vi "Set Support Directory.vi"(8 "error in (no error)":errorcluster, 10 "Support Directory Path":path, 11 "ProjectItem in":refnum<vi>) -> (0 "error out":errorcluster, 3 "ProjectItem out":refnum<vi>)   [LabVIEW 2019, in "Project Sync Tools.lvclass"]
uses:
  Project Sync Tools.lvclass
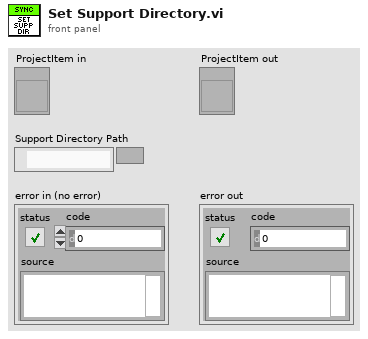
[diagram p1: front panel]
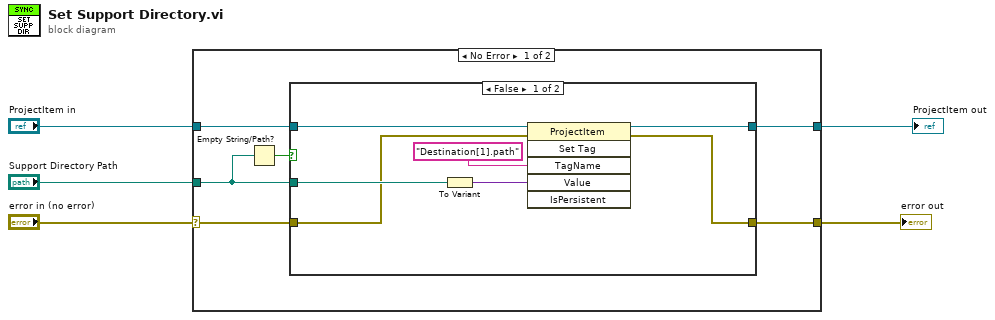
[diagram p0: block diagram]
diagram:
  n1 = case shown="No Error" "error in (no error)" {
    selector: "error in (no error)" -> [w8 w21]
    tunnel: [w11 w21] -> w5
    tunnel: [w10 w22] -> w4
    tunnel: "Support Directory Path" -> [w7 _]
    tunnel: "ProjectItem in" -> [w9 w22]
    frame No Error {
      n2 = Empty String/Path?(string/path=w7) -> (empty?=w6:bool)
      n3 = case shown="False" w6 {
        tunnel: [w18 w19] -> w11
        tunnel: [w17 w20] -> w10
        tunnel: w7 -> [w15 _]
        tunnel: w9 -> [w13 w20]
        tunnel: w8 -> [w12 w19]
        frame False {
          n4 = To Variant(anything=w15) -> (Variant=w16:variant)
          n5 = invoke class="ProjectItem" method="Set Tag"(reference=w13, error in=w12, "TagName"="Destination[1].path" ("Tag Name"), "Value"=w16) -> (reference out=w17:refnum<vi>, error out=w18:errorcluster)  [unwired: 2 in, 4 out]
        }
        frame True {
        }
      }
    }
    frame Error {
    }
  }
  "error out" <- w5
  "ProjectItem out" <- w4
